vi "Stages Messenger.vi"(0 "Stage Notifier Name":string="ProScan3", 2 "Actions":T2, 5 "Setpoint":dbl[](array[numeric]), 7 "Axis":bool[](array[boolean]), 9 "Velocity":dbl, 11 "Misc":variant, 13 "Exit While Busy?":bool) -> (4 "Stage Notifier Name (Dup)":string, 6 "Positions":dbl[](array[numeric]), 8 "Status":T1, 15 "Error":errorcluster)   [LabVIEW 2016]
uses:
  Stages Controls/Stage Actions.ctl
  Stages Controls/Stage Status.ctl
  Stages Controls/Stage Notifier Element.ctl
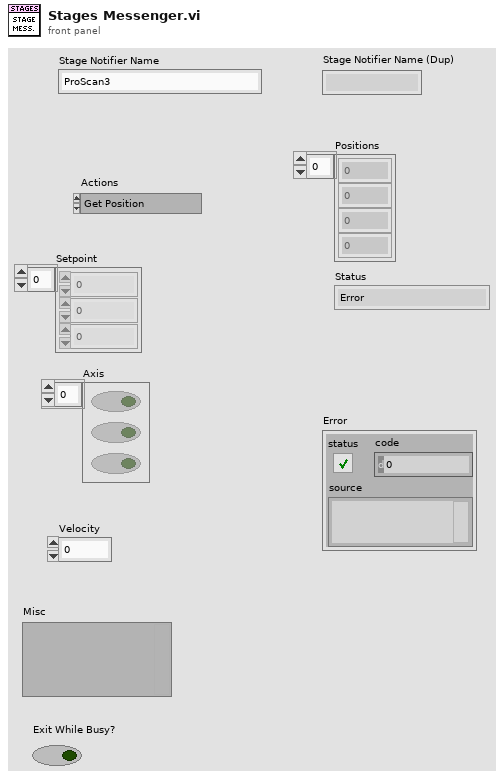
[diagram p1: front panel]
types:
  T1 = typedef "Stage Status.ctl" = enum16{"Error", "Abort", "Busy", "On Target"}
  T2 = typedef "Stage Actions.ctl" = enum16{"Get Position", "MVR", "SVR", "MOVE", "SVA", "HALT", "ONTARGET", "ERROR", "REFERENCE", "INIT", "VELOCITY", "STATUS", "EXIT", "HOME", "ZEROPOS", "NANOPOS", "ANALOG", "QUIT"}
  T3 = typedef "Stage Notifier Element.ctl" = cluster{"Action":T2, "Axis":bool[], "Setpoint":dbl[], "Velocity":dbl, "Cmd Recvd?":bool, "Position":dbl[], "Status":T1, "Misc":variant}
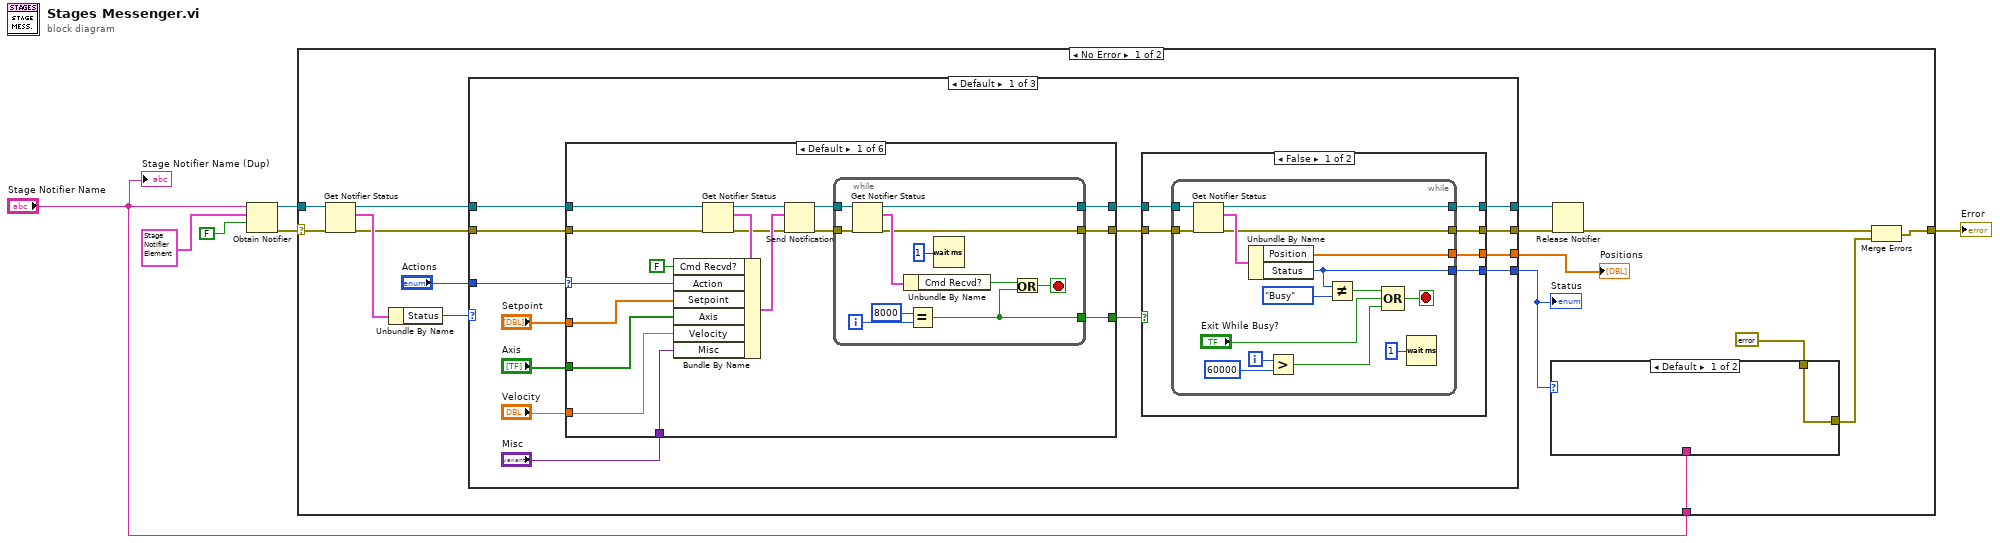
[diagram p0: block diagram]
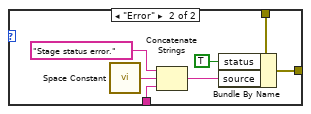
[diagram p2: hidden frame]
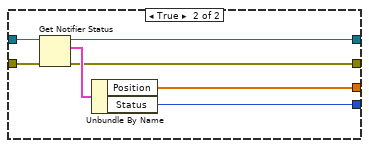
[diagram p3: hidden frame]
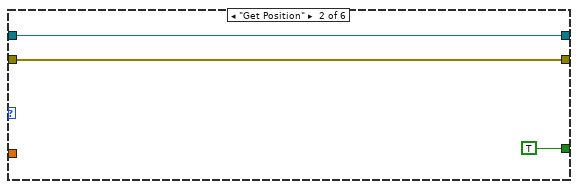
[diagram p4: hidden frame]
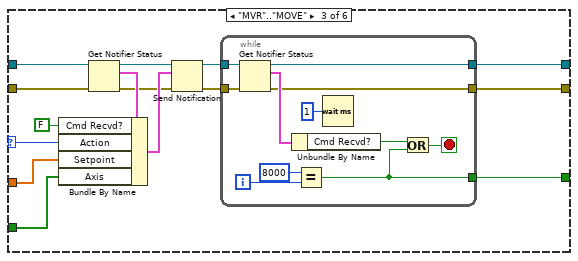
[diagram p5: hidden frame]
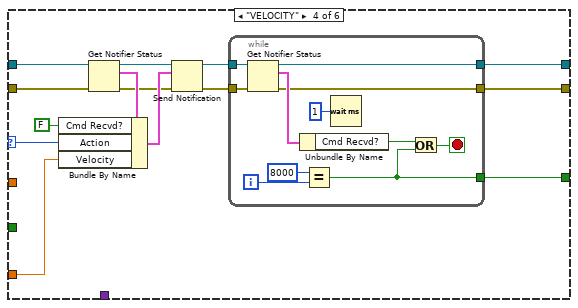
[diagram p6: hidden frame]
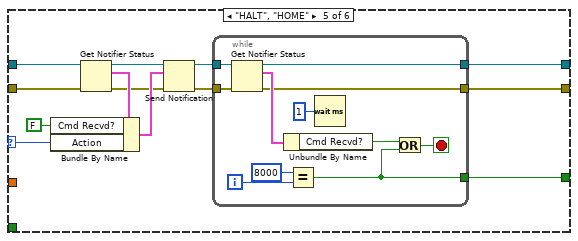
[diagram p7: hidden frame]
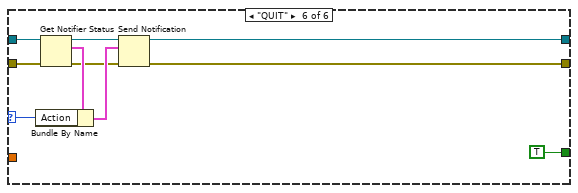
[diagram p8: hidden frame]
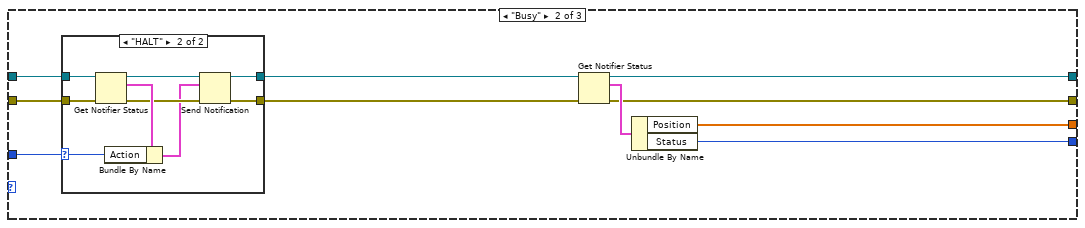
[diagram p9: hidden frame]
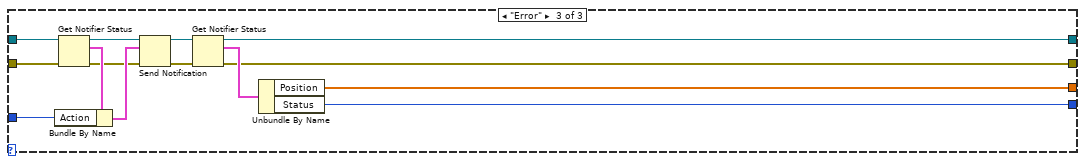
[diagram p11: hidden frame]
diagram:
  n1 = Obtain Notifier(name (unnamed)="Stage Notifier Name", notification data type=T3 {"Action"=enum."Get Position", "Axis"=[], "Setpoint"=[], "Velocity"=0.5, "Cmd Recvd?"=FALSE, "Position"=[], "Status"=enum."Error", "Misc"=variant} ("Stage Status"), create if not found? (T)=FALSE) -> (notifier out=w3:refnum<notifier>, error out=w4:errorcluster)  [unwired: 1 in, 1 out]
  n2 = case shown="No Error" w4 {
    selector: w4 -> [w16 w224]
    tunnel: w3 -> [w22 _]
    tunnel: "Stage Notifier Name" -> [w11 _]
    tunnel: [w8 w224] -> w1
    frame No Error {
      n3 = Get Notifier Status(notifier=w22, error in (no error)=w16) -> (notifier out=w20:refnum<notifier>, current notification=w21:T3, error out=w15:errorcluster)  [unwired: 2 out]
      n4 = Unbundle By Name(w21) -> ("Status"=w13:T1)
      n5 = case shown="Default" w13 {
        tunnel: w20 -> [w44 w192 w223]
        tunnel: [w37 w197 w217] -> w19
        tunnel: [w36 w196 w216] -> w18
        tunnel: [w35 w195 w215] -> w12
        tunnel: "Actions" -> [w43 w193 w221]
        tunnel: w15 -> [w34 w191 w213]
        tunnel: [w32 w194 w210] -> w14
        frame Default {
          n6 = case shown="Default" w43 {
            selector: w43 -> [w85 _ w114 w139 w163 w184]
            tunnel: w44 -> [w86 w103 w115 w140 w164 w187]
            tunnel: [w78 w103 w109 w136 w160 w188] -> w38
            tunnel: "Setpoint" -> [w82 _ w111 _ _ _]
            tunnel: "Axis" -> [w81 _ w110 _ _ _]
            tunnel: "Velocity" -> [w80 _ _ w130 _ _]
            tunnel: "Misc" -> [w79 _ _ _ _ _]
            tunnel: [w77 TRUE w108 w135 w159 TRUE] -> w39
            tunnel: w34 -> [w76 w102 w107 w134 w158 w181]
            tunnel: [w73 w102 w104 w131 w155 w179] -> w33
            frame Default {
              n7 = Get Notifier Status(notifier=w86, error in (no error)=w76) -> (notifier out=w87:refnum<notifier>, current notification=w88:T3, error out=w75:errorcluster)  [unwired: 2 out]
              n8 = Bundle By Name(cluster=w88, "Cmd Recvd?"=FALSE, "Action"=w85, "Setpoint"=w82, "Axis"=w81, "Velocity"=w80, "Misc"=w79) -> (w89:T3)
              n9 = Send Notification(notification=w89, notifier=w87, error in (no error)=w75) -> (notifier out=w83:refnum<notifier>, error out=w74:errorcluster)
              n10 = while {
                tunnel: w83 -> [w100]
                tunnel: [w97] -> w78
                tunnel: [w93] -> w77
                tunnel: w74 -> [w91]
                tunnel: [w90] -> w73
                i -> [w96]
                stop <- w92 stop-if-true
                n11 = Get Notifier Status(notifier=w100, error in (no error)=w91) -> (notifier out=w97:refnum<notifier>, current notification=w99:T3, error out=w90:errorcluster)  [unwired: 2 out]
                n12 = Unbundle By Name(w99) -> ("Cmd Recvd?"=w94:bool)
                n13 = Equal?(x=8000, y=w96) -> (x = y?=w93:bool)
                n14 = Wait (ms)(milliseconds to wait=u32 1) -> ()  [unwired: 1 out]
                n15 = Or(x=w94, y=w93) -> (x .or. y?=w92:bool)
              }
            }
            frame "Get Position" {
            }
            frame "MVR".."MOVE" {
              n16 = Get Notifier Status(notifier=w115, error in (no error)=w107) -> (notifier out=w116:refnum<notifier>, current notification=w117:T3, error out=w106:errorcluster)  [unwired: 2 out]
              n17 = Bundle By Name(cluster=w117, "Cmd Recvd?"=FALSE, "Action"=w114, "Setpoint"=w111, "Axis"=w110) -> (w118:T3)
              n18 = Send Notification(notification=w118, notifier=w116, error in (no error)=w106) -> (notifier out=w112:refnum<notifier>, error out=w105:errorcluster)
              n19 = while {
                tunnel: w112 -> [w129]
                tunnel: [w126] -> w109
                tunnel: [w122] -> w108
                tunnel: w105 -> [w120]
                tunnel: [w119] -> w104
                i -> [w125]
                stop <- w121 stop-if-true
                n20 = Get Notifier Status(notifier=w129, error in (no error)=w120) -> (notifier out=w126:refnum<notifier>, current notification=w128:T3, error out=w119:errorcluster)  [unwired: 2 out]
                n21 = Unbundle By Name(w128) -> ("Cmd Recvd?"=w123:bool)
                n22 = Equal?(x=8000, y=w125) -> (x = y?=w122:bool)
                n23 = Wait (ms)(milliseconds to wait=u32 1) -> ()  [unwired: 1 out]
                n24 = Or(x=w123, y=w122) -> (x .or. y?=w121:bool)
              }
            }
            frame "VELOCITY" {
              n25 = Get Notifier Status(notifier=w140, error in (no error)=w134) -> (notifier out=w141:refnum<notifier>, current notification=w142:T3, error out=w133:errorcluster)  [unwired: 2 out]
              n26 = Bundle By Name(cluster=w142, "Cmd Recvd?"=FALSE, "Action"=w139, "Velocity"=w130) -> (w143:T3)
              n27 = Send Notification(notification=w143, notifier=w141, error in (no error)=w133) -> (notifier out=w137:refnum<notifier>, error out=w132:errorcluster)
              n28 = while {
                tunnel: w137 -> [w154]
                tunnel: [w151] -> w136
                tunnel: [w147] -> w135
                tunnel: w132 -> [w145]
                tunnel: [w144] -> w131
                i -> [w150]
                stop <- w146 stop-if-true
                n29 = Get Notifier Status(notifier=w154, error in (no error)=w145) -> (notifier out=w151:refnum<notifier>, current notification=w153:T3, error out=w144:errorcluster)  [unwired: 2 out]
                n30 = Unbundle By Name(w153) -> ("Cmd Recvd?"=w148:bool)
                n31 = Equal?(x=8000, y=w150) -> (x = y?=w147:bool)
                n32 = Wait (ms)(milliseconds to wait=u32 1) -> ()  [unwired: 1 out]
                n33 = Or(x=w148, y=w147) -> (x .or. y?=w146:bool)
              }
            }
            frame "HALT", "HOME" {
              n34 = Get Notifier Status(notifier=w164, error in (no error)=w158) -> (notifier out=w165:refnum<notifier>, current notification=w166:T3, error out=w157:errorcluster)  [unwired: 2 out]
              n35 = Bundle By Name(cluster=w166, "Cmd Recvd?"=FALSE, "Action"=w163) -> (w167:T3)
              n36 = Send Notification(notification=w167, notifier=w165, error in (no error)=w157) -> (notifier out=w161:refnum<notifier>, error out=w156:errorcluster)
              n37 = while {
                tunnel: w161 -> [w178]
                tunnel: [w175] -> w160
                tunnel: [w171] -> w159
                tunnel: w156 -> [w169]
                tunnel: [w168] -> w155
                i -> [w174]
                stop <- w170 stop-if-true
                n38 = Get Notifier Status(notifier=w178, error in (no error)=w169) -> (notifier out=w175:refnum<notifier>, current notification=w177:T3, error out=w168:errorcluster)  [unwired: 2 out]
                n39 = Unbundle By Name(w177) -> ("Cmd Recvd?"=w172:bool)
                n40 = Equal?(x=8000, y=w174) -> (x = y?=w171:bool)
                n41 = Wait (ms)(milliseconds to wait=u32 1) -> ()  [unwired: 1 out]
                n42 = Or(x=w172, y=w171) -> (x .or. y?=w170:bool)
              }
            }
            frame "QUIT" {
              n43 = Get Notifier Status(notifier=w187, error in (no error)=w181) -> (notifier out=w186:refnum<notifier>, current notification=w185:T3, error out=w180:errorcluster)  [unwired: 2 out]
              n44 = Bundle By Name(cluster=w185, "Action"=w184) -> (w183:T3)
              n45 = Send Notification(notification=w183, notifier=w186, error in (no error)=w180) -> (notifier out=w188:refnum<notifier>, error out=w179:errorcluster)
            }
          }
          n46 = case shown="False" w39 {
            tunnel: w38 -> [w50 w72]
            tunnel: [w49 w71] -> w37
            tunnel: [w48 w70] -> w36
            tunnel: [w47 w68] -> w35
            tunnel: w33 -> [w46 w67]
            tunnel: [w45 w66] -> w32
            frame False {
              n47 = while {
                tunnel: w50 -> [w65]
                tunnel: [w64] -> w49
                tunnel: [w62] -> w48
                tunnel: [w56] -> w47
                tunnel: w46 -> [w52]
                tunnel: [w51] -> w45
                i -> [w58]
                stop <- w53 stop-if-true
                n48 = Get Notifier Status(notifier=w65, error in (no error)=w52) -> (notifier out=w64:refnum<notifier>, current notification=w63:T3, error out=w51:errorcluster)  [unwired: 2 out]
                n49 = Unbundle By Name(w63) -> ("Position"=w62:dbl[], "Status"=w56:T1)
                n50 = Greater?(x=w58, y=60000) -> (0:w54:bool)
                n51 = Not Equal?(x=w56, y=Stage_Status."Busy") -> (x != y?=w59:bool)
                n52 = Compound Arithmetic op=OR(w59, "Exit While Busy?", w54) -> (w53:bool)
                n53 = Wait (ms)(milliseconds to wait=u32 1) -> ()  [unwired: 1 out]
              }
            }
            frame True {
              n54 = Get Notifier Status(notifier=w72, error in (no error)=w67) -> (notifier out=w71:refnum<notifier>, current notification=w69:T3, error out=w66:errorcluster)  [unwired: 2 out]
              n55 = Unbundle By Name(w69) -> ("Position"=w70:dbl[], "Status"=w68:T1)
            }
          }
        }
        frame "Busy" {
          n56 = case shown="\"HALT\"" w193 {
            selector: w193 -> [_ w206]
            tunnel: w192 -> [w200 w209]
            tunnel: w191 -> [w199 w208]
            tunnel: [w200 w203] -> w190
            tunnel: [w199 w202] -> w189
            frame Default {
            }
            frame "HALT" {
              n57 = Get Notifier Status(notifier=w209, error in (no error)=w208) -> (notifier out=w205:refnum<notifier>, current notification=w207:T3, error out=w204:errorcluster)  [unwired: 2 out]
              n58 = Bundle By Name(cluster=w207, "Action"=w206) -> (w201:T3)
              n59 = Send Notification(notification=w201, notifier=w205, error in (no error)=w204) -> (notifier out=w203:refnum<notifier>, error out=w202:errorcluster)
            }
          }
          n60 = Get Notifier Status(notifier=w190, error in (no error)=w189) -> (notifier out=w197:refnum<notifier>, current notification=w198:T3, error out=w194:errorcluster)  [unwired: 2 out]
          n61 = Unbundle By Name(w198) -> ("Position"=w196:dbl[], "Status"=w195:T1)
        }
        frame "Error" {
          n62 = Get Notifier Status(notifier=w223, error in (no error)=w213) -> (notifier out=w220:refnum<notifier>, current notification=w222:T3, error out=w212:errorcluster)  [unwired: 2 out]
          n63 = Bundle By Name(cluster=w222, "Action"=w221) -> (w219:T3)
          n64 = Send Notification(notification=w219, notifier=w220, error in (no error)=w212) -> (notifier out=w218:refnum<notifier>, error out=w211:errorcluster)
          n65 = Get Notifier Status(notifier=w218, error in (no error)=w211) -> (notifier out=w217:refnum<notifier>, current notification=w214:T3, error out=w210:errorcluster)  [unwired: 2 out]
          n66 = Unbundle By Name(w214) -> ("Position"=w216:dbl[], "Status"=w215:T1)
        }
      }
      "Positions" <- w18
      "Status" <- w12
      n67 = case shown="Default" w12 {
        tunnel: w11 -> [_ w27]
        tunnel: [w23 w25] -> w9
        tunnel: errorcluster {"status"=FALSE, "code"=0, "source"=""} ("Error 2") -> [w23 w24]
        frame Default {
        }
        frame "Error" {
          n68 = call <vilib>:"Space Constant.vi"() -> ("String"=w28:string)
          n69 = Concatenate Strings("Stage status error." ("source"), w28, w27) -> (w26:string)
          n70 = Bundle By Name(cluster=w24, "status"=TRUE, "source"=w26) -> (w25:errorcluster)
        }
      }
      n71 = Release Notifier(notifier=w19, error in (no error)=w14) -> (error out=w10:errorcluster)  [unwired: 1 in, 2 out]
      n72 = Merge Errors(w10, w9) -> (w8:errorcluster)
    }
    frame Error {
    }
  }
  "Error" <- w1
  "Stage Notifier Name (Dup)" <- "Stage Notifier Name"
